vi "Translate Data.vi"(8 "error in (no error)":errorcluster, 10 "BufferIn":string, 11 "Alicat_P in":refnum<class "P.lvclass">) -> (0 "error out":errorcluster, 2 "DataOut":refnum<class "Data.lvclass">, 3 "Alicat_P out":refnum<class "P.lvclass">)   [LabVIEW 2014, in "Alicat.lvlib" / "P.lvclass"]
doc: "VI used to translate the data buffer to something meaningful (implementation dependent). This VI must be overridden."
uses:
  P.lvclass
  reusable/Data/Data.lvclass
  Data/P/AlicatPData.lvclass
  P.lvclass/P.ctl
  <vilib>/gmath/NI_Gmath.lvlib
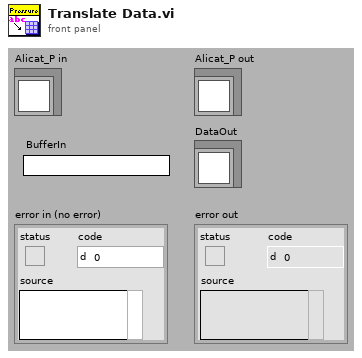
[diagram p1: front panel]
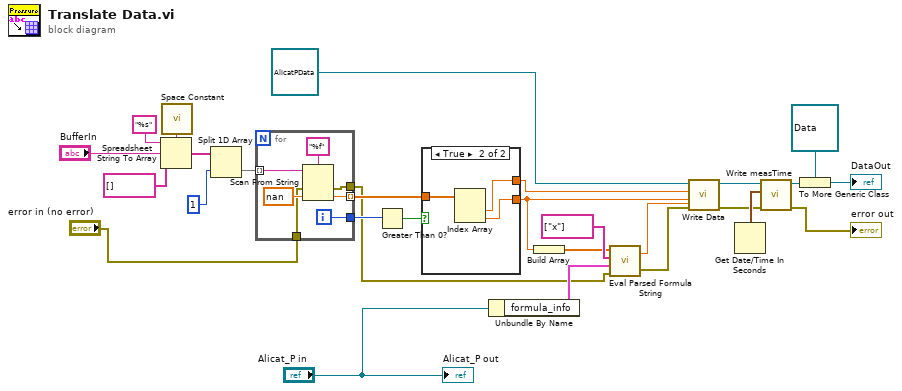
[diagram p0: block diagram]
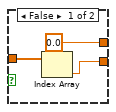
[diagram p2: hidden frame]
diagram:
  n1 = call <vilib>:"Space Constant.vi"() -> ("String"=w27:string)
  n2 = Spreadsheet String To Array(delimiter (Tab)=w27, format string="%s", spreadsheet string="BufferIn", array type (2D Dbl)=string[] []) -> (array=w24:string[])
  n3 = Split 1D Array(array=w24, index=1) -> (second subarray=w22:string[])  [unwired: 1 out]
  n4 = for {
    tunnel: w22 -> [w35] mode=indexing
    tunnel: [w32] -> w14 mode=indexing
    tunnel: "error in (no error)" -> [w31]
    tunnel: [w30] -> w2
    tunnel: [w29] -> w16
    i -> [w29]
    n5 = Scan From String(format string="%f", input string=w35, error in=w31, default 1=sgl nan ("default value 1")) -> (error out=w30:errorcluster, output 1=w32:sgl)  [unwired: 1 in, 2 out]
  }
  n6 = Greater Than 0?(x=w16) -> (x > 0?=w15:bool)
  n7 = case shown="True" w15 {
    tunnel: w14 -> [w38 w41]
    tunnel: [w37 w39] -> w5
    tunnel: [0.0 ("P") w40] -> w13
    frame False {
      n8 = Index Array(array=w38) -> (element=w37:sgl)  [unwired: 1 in]
    }
    frame True {
      n9 = Index Array(array=w41) -> (element #1=w40:sgl, element #2=w39:sgl)  [unwired: 2 in]
    }
  }
  n10 = Unbundle By Name("Alicat_P in") -> ("formula_info"=w7:cluster{"Table":i32[][], "Y Values":dbl[]})
  n11 = Build Array(w5) -> (w4:sgl[])
  n12 = call <vilib>:"Eval Parsed Formula String.vi"("error in (no error)"=w2, "Parsed Formula"=w7, "Variables"=string[] ["x"], "X Values"=w4) -> ("error out"=w1:errorcluster, "y value"=w3:dbl)
  n13 = call "Write Data.vi"("Q"=w3, "error in"=w1, "dP"=w5, "P"=w13, "AlicatPData in"=refnum<class "AlicatPData.lvclass"> refnum ("AlicatPData.lvclass")) -> ("error out"=w17:errorcluster, "AlicatPData out"=w18:refnum<class "AlicatPData.lvclass">)  [unwired: 5 in]
  n14 = Get Date/Time In Seconds() -> (seconds since 1Jan1904=w19:timestamp)
  n15 = call "Write measTime.vi"("error in (no error)"=w17, "measTime"=w19, "Data in"=w18) -> ("error out"=→"error out":errorcluster, "Data out"=w11:refnum<class "AlicatPData.lvclass">)  [unwired: 7 in]
  n16 = To More Generic Class(target class=refnum<class "Data.lvclass"> refnum ("DataOut"), reference=w11) -> (generic class reference=→"DataOut":refnum<class "Data.lvclass">)
  "Alicat_P out" <- "Alicat_P in"
